vi "Begin.vi"(8 "error in":errorcluster) -> (0 "error out":errorcluster)   [LabVIEW 2018]
doc: "Called before other user functions, this VI is expected to open initial I/O refnums, load in file data, and do all program initialization. Notice that the <B>error out</B> terminal is simply used for data flow. Wiring it to other structures or subVIs ensures that this VI runs first."
uses:
  <vilib>/Rock Robotics/WPI/ThirdParty/Phoenix-LabVIEW/Motor Controller/Controls/CTRE_Phoenix_MotorControl_EnhancedMotorControllerConfigurables.ctl
  <vilib>/Rock Robotics/WPI/ThirdParty/Phoenix-LabVIEW/Motor Controller/Controls/CTRE_Phoenix_MotorControl_BaseConfigurables.ctl
  <vilib>/Rock Robotics/WPI/ThirdParty/Phoenix-LabVIEW/Motor Controller/Controls/CTRE_Phoenix_MotorControl_VelocityMeasurementPeriod.ctl
  <vilib>/Rock Robotics/WPI/ThirdParty/Phoenix-LabVIEW/Motor Controller/Controls/CTRE_Phoenix_MotorControl_SlotStructure.ctl
  <vilib>/Rock Robotics/WPI/ThirdParty/Phoenix-LabVIEW/Motor Controller/Controls/CTRE_Phoenix_MotorControl_FilterStruct.ctl
  <vilib>/Rock Robotics/WPI/ThirdParty/Phoenix-LabVIEW/Motor Controller/Controls/CTRE_Phoenix_MotorControl_RemoteSourceType.ctl
  <vilib>/Rock Robotics/WPI/ThirdParty/Phoenix-LabVIEW/Controls/CTRE_Phoenix_CustomParamConfiguration.ctl
  <vilib>/Rock Robotics/WPI/ThirdParty/Phoenix-LabVIEW/Motor Controller/Controls/CTRE_Phoenix_MotorControl_FeedbackDevice.ctl
  <vilib>/Rock Robotics/WPI/ThirdParty/Phoenix-LabVIEW/Motor Controller/Controls/CTRE_Phoenix_MotorControl_SensorTermFeedbackDevice_Enhanced.ctl
  <vilib>/Rock Robotics/WPI/ThirdParty/Phoenix-LabVIEW/Motor Controller/Controls/CTRE_Phoenix_MotorControl_LimitSwitchNormal.ctl
  <vilib>/Rock Robotics/WPI/ThirdParty/Phoenix-LabVIEW/Motor Controller/Controls/CTRE_Phoenix_MotorControl_LimitSwitchSource_Local.ctl
  <vilib>/Rock Robotics/WPI/ThirdParty/Phoenix-LabVIEW/Motor Controller/Controls/CTRE_Phoenix_MotorControl_MotorControllerConfigurables.ctl
  <vilib>/Rock Robotics/WPI/ThirdParty/Phoenix-LabVIEW/Motor Controller/Controls/CTRE_Phoenix_MotorControl_RemoteFeedbackDevice.ctl
  <vilib>/Rock Robotics/WPI/ThirdParty/Phoenix-LabVIEW/Motor Controller/Controls/CTRE_Phoenix_MotorControl_SensorTermFeedbackDevice.ctl
  <vilib>/Rock Robotics/WPI/ThirdParty/Phoenix-LabVIEW/Motor Controller/Controls/CTRE_Phoenix_MotorControl_LimitSwitchSource.ctl
  <vilib>/Rock Robotics/WPI/DriverStation/WPI_DriverStationRobotMode2.ctl
  <vilib>/Rock Robotics/WPI/Joystick/WPI_JoystickDeviceEnum.ctl
  <vilib>/Rock Robotics/WPI/ThirdParty/REV Robotics/SPARK MAX/Typedef/Spark MAX Idle Mode.ctl
  <vilib>/Rock Robotics/WPI/ThirdParty/Phoenix-LabVIEW/Motor Controller/Controls/CTRE_Phoenix_MotorControl_NeutralMode.ctl
  <vilib>/Rock Robotics/WPI/Solenoid/WPI_SolenoidChannel.ctl
  <vilib>/Rock Robotics/SystemInterfaces/AI/FPGA_AIChannel.ctl
  <vilib>/Rock Robotics/WPI/Accelerometer/WPI_AccelerometerRange.ctl
  Robot Global Data.vi
  <vilib>/Rock Robotics/Network Tables/NT Write String Array.vi
  Joystick RefNum.vi
  RefNums_Actuators.vi
  CurrentMonitoring.vi
  <vilib>/Rock Robotics/WPI/Solenoid/WPI_SolenoidOpenDouble.vi
  <vilib>/Rock Robotics/WPI/Utilities/WPI_GetSetVariantRefNum.vi
  RefNums_Sensors.vi
  <vilib>/Rock Robotics/WPI/Accelerometer/InternalAccelerometer/WPI_AccelerometerInternalOpen.vi
  <vilib>/Rock Robotics/WPI/Solenoid/WPI_SolenoidOpenSingle.vi
  <vilib>/Rock Robotics/SystemInterfaces/DIO/FPGA_DIOPWMChannel.ctl
panel:
  in  "Victor Enhanced Control":T1={"Base Configurables"={"openLoopRamp"=0.0, "closedLoopRamp"=0.0, "peakOutputForward"=1.0, "peakOutputReverse"=-1.0, "nominalOutputForward"=0.0, "nominalOutputReverse"=0.0, "neutralDeadband"=0.04, "voltageCompSaturation"=0.0, "voltageMeasurementFilter"=32, "velocityMeasurementPeriod"=100, "velocityMeasurementWindow"=64, "forwardSoftLimitThreshold"=0, "reverseSoftLimitThreshold"=0, "forwardSoftLimitEnable"=FALSE, "reverseSoftLimitEnable"=FALSE, "slot0"={"P"=0.0, "I"=0.0, "D"=0.0, "F"=0.0, "integralZone"=0.0, "allowableClosedLoopError"=0, "maxIntegralAccumulator"=0.0, "closedLoopPeakOutput"=1.0, "closedLoopPeriod"=1}, "slot1"={"P"=0.0, "I"=0.0, "D"=0.0, "F"=0.0, "integralZone"=0.0, "allowableClosedLoopError"=0, "maxIntegralAccumulator"=0.0, "closedLoopPeakOutput"=1.0, "closedLoopPeriod"=1}, "slot2"={"P"=0.0, "I"=0.0, "D"=0.0, "F"=0.0, "integralZone"=0.0, "allowableClosedLoopError"=0, "maxIntegralAccumulator"=0.0, "closedLoopPeakOutput"=1.0, "closedLoopPeriod"=1}, "slot3"={"P"=0.0, "I"=0.0, "D"=0.0, "F"=0.0, "integralZone"=0.0, "allowableClosedLoopError"=0, "maxIntegralAccumulator"=0.0, "closedLoopPeakOutput"=1.0, "closedLoopPeriod"=1}, "auxPIDPolarity"=FALSE, "remoteFilter0"={"remoteSensorDeviceID"=0, "remoteSensorSource"=enum."Off"}, "remoteFilter1"={"remoteSensorDeviceID"=0, "remoteSensorSource"=enum."Off"}, "motionCruiseVelocity"=0, "motionAcceleration"=0, "motionProfileTrajectoryPeriod"=0, "feedbackNotContinuous"=FALSE, "remoteSensorClosedLoopDisableNeutralOnLOS"=FALSE, "clearPositionOnLimitF"=FALSE, "clearPositionOnLimitR"=FALSE, "clearPositionOnQuadIdx"=FALSE, "limitSwitchDisableNeutralOnLOS"=FALSE, "softLimitDisableNeutralOnLOS"=FALSE, "pulseWidthPeriod_EdgesPerRot"=1, "pulseWidthPeriod_FilterWindowSz"=1, "customParam"={"customParam0"=0, "customParam1"=0}, "trajectoryInterpolationEnable"=TRUE}, "primaryPID"={"selectedFeedbackCoefficient"=1.0, "selectedFeedbackSensor"=11}, "auxiliaryPID"={"selectedFeedbackCoefficient"=1.0, "selectedFeedbackSensor"=11}, "sum 0 term"=11, "sum 1 term"=11, "diff 0 term "=11, "diff 1 term"=11, "forwardLimitSwitchDeviceID"=0, "reverseLimitSwitchDeviceID"=0, "forwardLimitSwitchNormal"=enum."Normally Open", "reverseLimitSwitchNormal"=enum."Normally Open", "forwardLimitSwitchSource"=3, "reverseLimitSwitchSource"=3} {"diff 1 term" items=["Remote Source 0"=11, "Remote Source 1"=12, "Software Emulated"=15]; "diff 0 term" items=["Remote Source 0"=11, "Remote Source 1"=12, "Software Emulated"=15]; "sum 1 term" items=["Remote Source 0"=11, "Remote Source 1"=12, "Software Emulated"=15]; "sum 0 term" items=["Remote Source 0"=11, "Remote Source 1"=12, "Software Emulated"=15]; "reverseLimitSwitchSource" items=["Remote Talon SRX"=1, "Remote CANifier"=2, "Deactivated"=3]; "forwardLimitSwitchSource" items=["Remote Talon SRX"=1, "Remote CANifier"=2, "Deactivated"=3]; "auxiliaryPID"."selectedFeedbackSensor" items=["Sensor Sum (S0 + S1)"=9, "Sensor Difference (D0 - D1)"=10, "Remote Source 0"=11, "Remote Source 1"=12, "Software Emulated"=15]; "primaryPID"."selectedFeedbackSensor" items=["Sensor Sum (S0 + S1)"=9, "Sensor Difference (D0 - D1)"=10, "Remote Source 0"=11, "Remote Source 1"=12, "Software Emulated"=15]; "Base Configurables"."velocityMeasurementPeriod" items=["Period_1ms"=1, "Period_2ms"=2, "Period_5ms"=5, "Period_10ms"=10, "Period_20ms"=20, "Period_25ms"=25, "Period_50ms"=50, "Period_100ms"=100]}
  in  "Talon Enhanced Config":T12={"Base Configurables"={"openLoopRamp"=0.0, "closedLoopRamp"=0.0, "peakOutputForward"=1.0, "peakOutputReverse"=-1.0, "nominalOutputForward"=0.0, "nominalOutputReverse"=0.0, "neutralDeadband"=0.04, "voltageCompSaturation"=0.0, "voltageMeasurementFilter"=32, "velocityMeasurementPeriod"=100, "velocityMeasurementWindow"=64, "forwardSoftLimitThreshold"=0, "reverseSoftLimitThreshold"=0, "forwardSoftLimitEnable"=FALSE, "reverseSoftLimitEnable"=FALSE, "slot0"={"P"=0.0, "I"=0.0, "D"=0.0, "F"=0.0, "integralZone"=0.0, "allowableClosedLoopError"=0, "maxIntegralAccumulator"=0.0, "closedLoopPeakOutput"=1.0, "closedLoopPeriod"=1}, "slot1"={"P"=0.0, "I"=0.0, "D"=0.0, "F"=0.0, "integralZone"=0.0, "allowableClosedLoopError"=0, "maxIntegralAccumulator"=0.0, "closedLoopPeakOutput"=1.0, "closedLoopPeriod"=1}, "slot2"={"P"=0.0, "I"=0.0, "D"=0.0, "F"=0.0, "integralZone"=0.0, "allowableClosedLoopError"=0, "maxIntegralAccumulator"=0.0, "closedLoopPeakOutput"=1.0, "closedLoopPeriod"=1}, "slot3"={"P"=0.0, "I"=0.0, "D"=0.0, "F"=0.0, "integralZone"=0.0, "allowableClosedLoopError"=0, "maxIntegralAccumulator"=0.0, "closedLoopPeakOutput"=1.0, "closedLoopPeriod"=1}, "auxPIDPolarity"=FALSE, "remoteFilter0"={"remoteSensorDeviceID"=0, "remoteSensorSource"=enum."Off"}, "remoteFilter1"={"remoteSensorDeviceID"=0, "remoteSensorSource"=enum."Off"}, "motionCruiseVelocity"=0, "motionAcceleration"=0, "motionProfileTrajectoryPeriod"=0, "feedbackNotContinuous"=FALSE, "remoteSensorClosedLoopDisableNeutralOnLOS"=FALSE, "clearPositionOnLimitF"=FALSE, "clearPositionOnLimitR"=FALSE, "clearPositionOnQuadIdx"=FALSE, "limitSwitchDisableNeutralOnLOS"=FALSE, "softLimitDisableNeutralOnLOS"=FALSE, "pulseWidthPeriod_EdgesPerRot"=1, "pulseWidthPeriod_FilterWindowSz"=1, "customParam"={"customParam0"=0, "customParam1"=0}, "trajectoryInterpolationEnable"=TRUE}, "primaryPID"={"selectedFeedbackCoefficient"=1.0, "selectedFeedbackSensor"=0}, "auxiliaryPID"={"selectedFeedbackCoefficient"=1.0, "selectedFeedbackSensor"=0}, "sum0Term"=0, "sum1Term"=0, "diff0Term"=0, "diff1Term"=0, "forwardLimitSwitchNormal"=enum."Normally Open", "reverseLimitSwitchNormal"=enum."Normally Open", "forwardLimitSwitchDeviceID"=0, "reverseLimitSwitchDeviceID"=0, "forwardLimitSwitchSource"=enum."Feedback Connector", "reverseLimitSwitchSource"=enum."Feedback Connector", "peakCurrentLimit"=1, "peakCurrentDuration"=1, "continuousCurrentLimit"=1} {"diff1Term" items=["QuadEncoder"=0, "Analog"=2, "Tachometer"=4, "Pulse Width Encoded Position"=8, "Remote Source 0"=11, "Remote Source 1"=12, "Software Emulated"=15]; "diff0Term" items=["QuadEncoder"=0, "Analog"=2, "Tachometer"=4, "Pulse Width Encoded Position"=8, "Remote Source 0"=11, "Remote Source 1"=12, "Software Emulated"=15]; "sum1Term" items=["QuadEncoder"=0, "Analog"=2, "Tachometer"=4, "Pulse Width Encoded Position"=8, "Remote Source 0"=11, "Remote Source 1"=12, "Software Emulated"=15]; "sum0Term" items=["QuadEncoder"=0, "Analog"=2, "Tachometer"=4, "Pulse Width Encoded Position"=8, "Remote Source 0"=11, "Remote Source 1"=12, "Software Emulated"=15]; "auxiliaryPID"."selectedFeedbackSensor" items=["QuadEncoder"=0, "Analog"=2, "Tachometer"=4, "Pulse Width Encoded Position"=8, "Sensor Sum (S0 + S1)"=9, "Sensor Difference (D0 - D1)"=10, "Remote Source 0"=11, "Remote Source 1"=12, "Software Emulated"=15]; "primaryPID"."selectedFeedbackSensor" items=["QuadEncoder"=0, "Analog"=2, "Tachometer"=4, "Pulse Width Encoded Position"=8, "Sensor Sum (S0 + S1)"=9, "Sensor Difference (D0 - D1)"=10, "Remote Source 0"=11, "Remote Source 1"=12, "Software Emulated"=15]; "Base Configurables"."velocityMeasurementPeriod" items=["Period_1ms"=1, "Period_2ms"=2, "Period_5ms"=5, "Period_10ms"=10, "Period_20ms"=20, "Period_25ms"=25, "Period_50ms"=50, "Period_100ms"=100]}
  # "Sum and Diff terms are ways to select more than one sensor as a feedback device. \n Sum 0 is the first feedback device to be used for the Sum term, \n Sum 1 is the feedback device to be added to Sum 0 for the Sum term\n Diff 0 and Diff 1 work in a similar manner"
  # "These are only applicable\nif using a remote limit switch.\n\nLocal limit switches/no limit\nswitches do not use this"
  # "False: Primary Output = PID[0] + PID[1]  ---  Auxiliary Output = PID[0] - PID[1]\nTrue:  Primary Output = PID[0] - PID[1] --- Auxiliary Output = PID[0] + PID[1]"
  # "Enable the motion profile executor to perform linear interpolation between profile points.  Defaults to True."
  # "Sum and Diff terms are ways to select more than one sensor as a feedback device. \n Sum 0 is the first feedback device to be used for the Sum term.\n Sum 1 is the feedback device to be added to Sum 0 for the Sum term.\n Diff 0 and Diff 1 work in a similar manner."
  # "These are only applicable\nif using a remote limit switch.\n\nLocal limit switches/no limit\nswitches do not use this."
  # "Current is below Continuous threshold AND\n\n(Requested output is weaker** than applied motor\noutput OR is in the opposite direction).\n/\nMotor output is set to requested output."
  # "Current is above Peak* Threshold for Peak Duration.\n/\nReduce motor output (towards neutral)."
  # "Current is below Continuous threshold.\n/\nRamp motor output towards requested output."
  # "Current is above Continuous threshold.\n/\nReduce motor output (towards neutral)."
  # "Current Limiting is NOT enabled\nby default.\nCall this VI to enable."
  # "*If the configured Peak Threshold is less than the Continuous Threshold, the applied Peak Threshold is set equal to the Configured Continuous Threshold in firmware.\n** Both requested output and applied motor output are in the same direction, and requested output is closer to neutral."
  # "False: Primary Output = PID[0] + PID[1]  ---  Auxiliary Output = PID[0] - PID[1]\nTrue:  Primary Output = PID[0] - PID[1] --- Auxiliary Output = PID[0] + PID[1]"
  # "Enable the motion profile executor to perform linear interpolation between profile points.  Defaults to True."
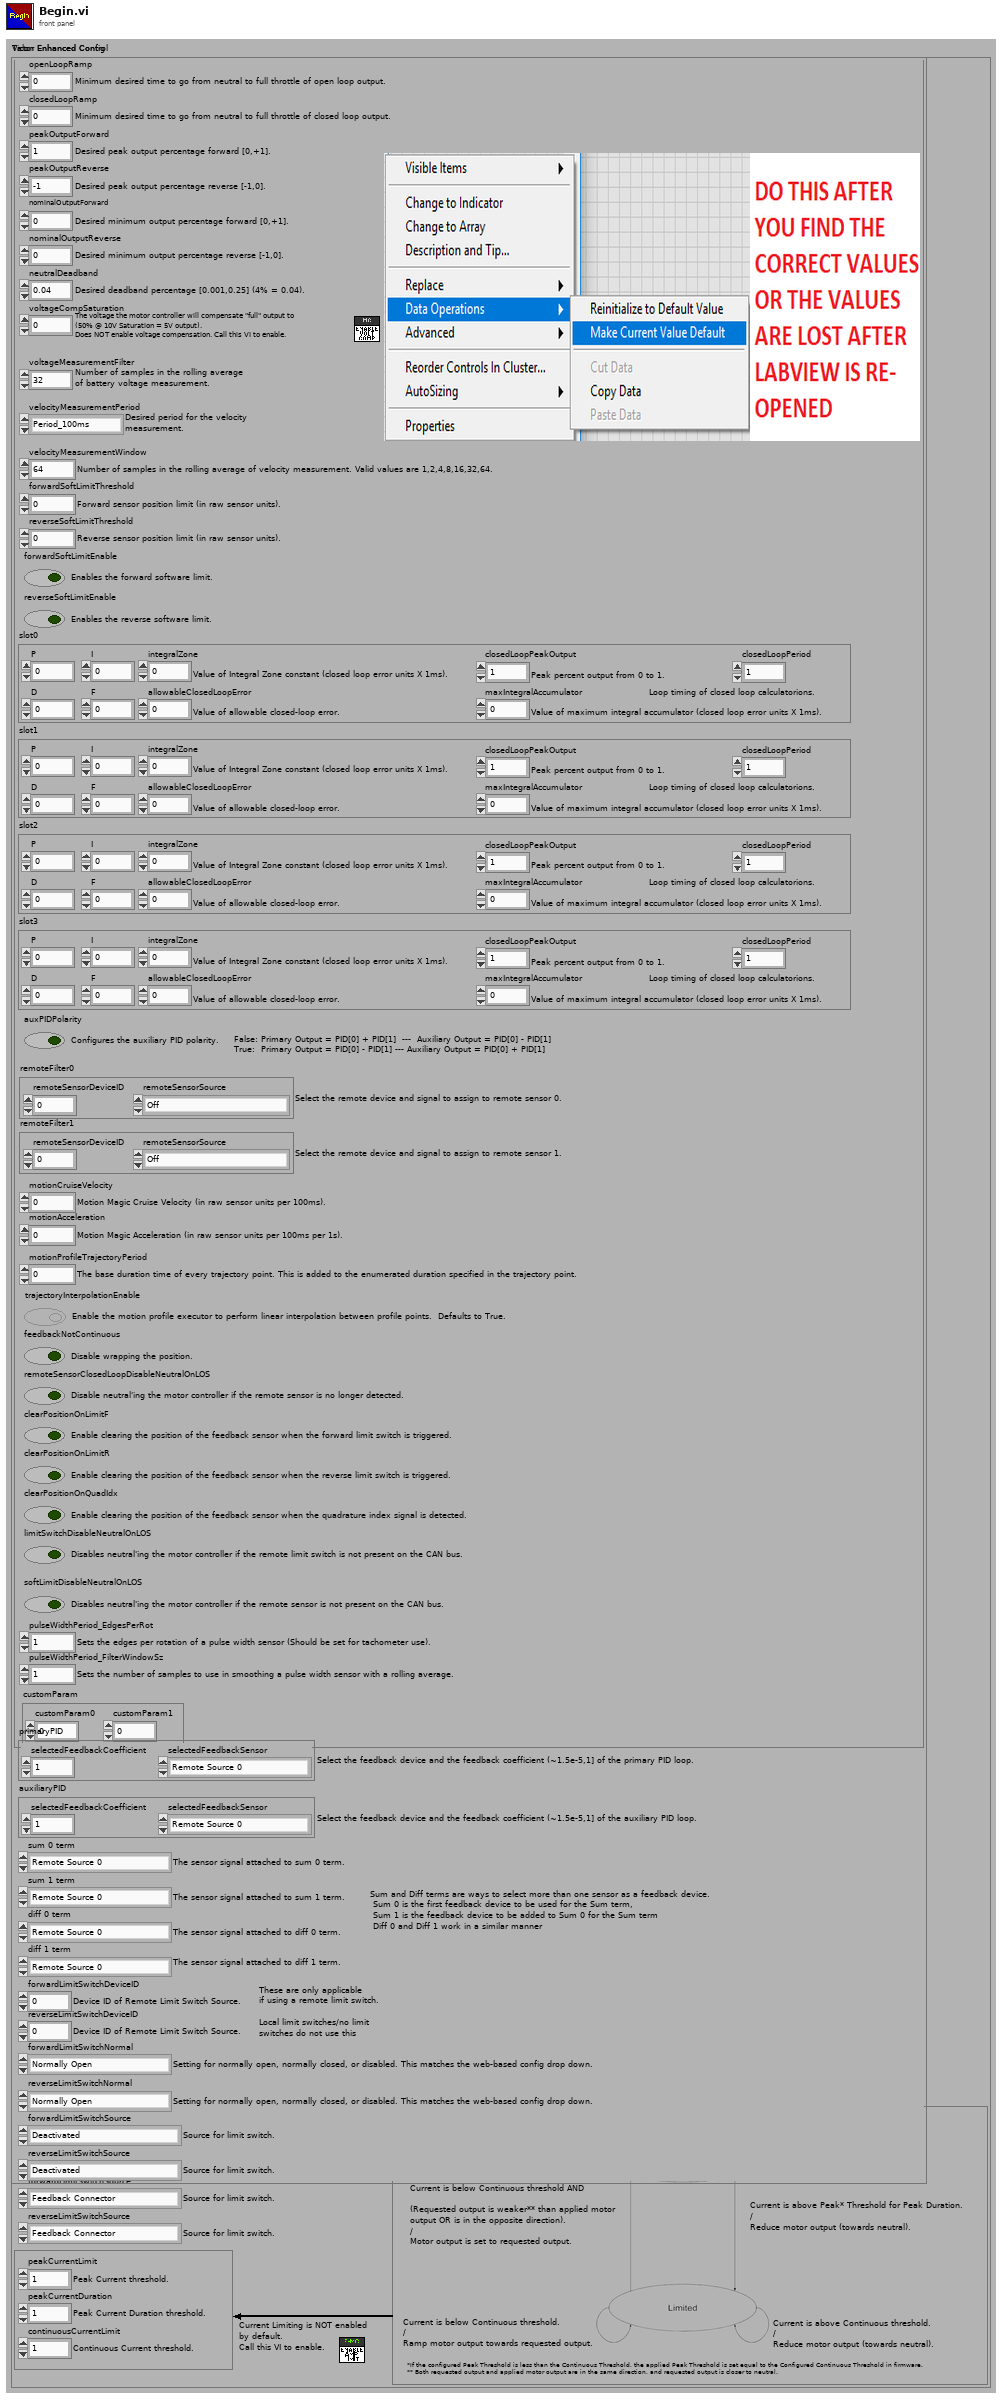
[diagram p1: front panel]
types:
  T1 = typedef "CTRE_Phoenix_MotorControl_MotorControllerConfigurables.ctl" = cluster{"Base Configurables":T2, "primaryPID":cluster{"selectedFeedbackCoefficient":dbl, "selectedFeedbackSensor":T8}, "auxiliaryPID":cluster{"selectedFeedbackCoefficient":dbl, "selectedFeedbackSensor":T8}, "sum 0 term":T9, "sum 1 term":T9, "diff 0 term ":T9, "diff 1 term":T9, "forwardLimitSwitchDeviceID":i32, "reverseLimitSwitchDeviceID":i32, "forwardLimitSwitchNormal":T10, "reverseLimitSwitchNormal":T10, "forwardLimitSwitchSource":T11, "reverseLimitSwitchSource":T11}
  T2 = typedef "CTRE_Phoenix_MotorControl_BaseConfigurables.ctl" = cluster{"openLoopRamp":dbl, "closedLoopRamp":dbl, "peakOutputForward":dbl, "peakOutputReverse":dbl, "nominalOutputForward":dbl, "nominalOutputReverse":dbl, "neutralDeadband":dbl, "voltageCompSaturation":dbl, "voltageMeasurementFilter":i32, "velocityMeasurementPeriod":T3, "velocityMeasurementWindow":i32, "forwardSoftLimitThreshold":i32, "reverseSoftLimitThreshold":i32, "forwardSoftLimitEnable":bool, "reverseSoftLimitEnable":bool, "slot0":T4, "slot1":T4, "slot2":T4, "slot3":T4, "auxPIDPolarity":bool, "remoteFilter0":T5, "remoteFilter1":T5, "motionCruiseVelocity":i32, "motionAcceleration":i32, "motionProfileTrajectoryPeriod":i32, "feedbackNotContinuous":bool, "remoteSensorClosedLoopDisableNeutralOnLOS":bool, "clearPositionOnLimitF":bool, "clearPositionOnLimitR":bool, "clearPositionOnQuadIdx":bool, "limitSwitchDisableNeutralOnLOS":bool, "softLimitDisableNeutralOnLOS":bool, "pulseWidthPeriod_EdgesPerRot":i32, "pulseWidthPeriod_FilterWindowSz":i32, "customParam":T7, "trajectoryInterpolationEnable":bool}
  T3 = typedef "CTRE_Phoenix_MotorControl_VelocityMeasurementPeriod.ctl" = u16
  T4 = typedef "CTRE_Phoenix_MotorControl_SlotStructure.ctl" = cluster{"P":dbl, "I":dbl, "D":dbl, "F":dbl, "integralZone":dbl, "allowableClosedLoopError":i32, "maxIntegralAccumulator":dbl, "closedLoopPeakOutput":dbl, "closedLoopPeriod":i32}
  T5 = typedef "CTRE_Phoenix_MotorControl_FilterStruct.ctl" = cluster{"remoteSensorDeviceID":u8, "remoteSensorSource":T6}
  T6 = typedef "CTRE_Phoenix_MotorControl_RemoteSourceType.ctl" = enum16{"Off", "Talon SRX Selected Sensor", "Pigeon IMU Yaw", "Pigeon IMU Pitch", "Pigeon IMU Roll", "CANifier Quadrature", "CANifier PWM Input 0", "CANifier PWM Input 1", "CANifier PWM Input 2", "CANifier PWM Input 3", "Gadgeteer Pigeon Yaw", "Gadgeteer Pigeon Pitch", "Gadgeteer Pigeon Roll"}
  T7 = typedef "CTRE_Phoenix_CustomParamConfiguration.ctl" = cluster{"customParam0":i32, "customParam1":i32}
  T8 = typedef "CTRE_Phoenix_MotorControl_RemoteFeedbackDevice.ctl" = i8
  T9 = typedef "CTRE_Phoenix_MotorControl_SensorTermFeedbackDevice.ctl" = i8
  T10 = typedef "CTRE_Phoenix_MotorControl_LimitSwitchNormal.ctl" = enum16{"Normally Open", "Normally Closed", "Disabled"}
  T11 = typedef "CTRE_Phoenix_MotorControl_LimitSwitchSource.ctl" = u16
  T12 = typedef "CTRE_Phoenix_MotorControl_EnhancedMotorControllerConfigurables.ctl" = cluster{"Base Configurables":T2, "primaryPID":cluster{"selectedFeedbackCoefficient":dbl, "selectedFeedbackSensor":T13}, "auxiliaryPID":cluster{"selectedFeedbackCoefficient":dbl, "selectedFeedbackSensor":T13}, "sum0Term":T14, "sum1Term":T14, "diff0Term":T14, "diff1Term":T14, "forwardLimitSwitchNormal":T10, "reverseLimitSwitchNormal":T10, "forwardLimitSwitchDeviceID":i32, "reverseLimitSwitchDeviceID":i32, "forwardLimitSwitchSource":T15, "reverseLimitSwitchSource":T15, "peakCurrentLimit":i32, "peakCurrentDuration":i32, "continuousCurrentLimit":i32}
  T13 = typedef "CTRE_Phoenix_MotorControl_FeedbackDevice.ctl" = i8
  T14 = typedef "CTRE_Phoenix_MotorControl_SensorTermFeedbackDevice_Enhanced.ctl" = i8
  T15 = typedef "CTRE_Phoenix_MotorControl_LimitSwitchSource_Local.ctl" = enum16{"Feedback Connector", "Remote Talon SRX", "Remote CANifier", "Deactivated"}
  T16 = typedef "WPI_AccelerometerRange.ctl" = enum16{"+/- 2 g", "+/- 4 g", "+/- 8 g"}
  T17 = typedef "FPGA_AIChannel.ctl" = enum8{"AI 0", "AI 1", "AI 2", "AI 3", "AI MXP 0", "AI MXP 1", "AI MXP 2", "AI MXP 3", "Invalid"}
  T18 = typedef "WPI_SolenoidChannel.ctl" = enum8{"Solenoid 0", "Solenoid 1", "Solenoid 2", "Solenoid 3", "Solenoid 4", "Solenoid 5", "Solenoid 6", "Solenoid 7", "Invalid"}
  T19 = typedef "CTRE_Phoenix_MotorControl_NeutralMode.ctl" = enum8{"EEPROMSetting", "Override to Coast", "Override to Brake"}
  T20 = typedef "Spark MAX Idle Mode.ctl" = enum16{"Coast", "Brake"}
  T21 = typedef "WPI_JoystickDeviceEnum.ctl" = enum16{"USB 0", "USB 1", "USB 2", "USB 3", "USB 4", "USB 5"}
  T22 = typedef "WPI_DriverStationRobotMode2.ctl" = enum16{"Autonomous Disabled", "Autonomous Enabled", "Teleop Disabled", "Teleop Enabled", "Disconnected", "Finish", "Test Disabled", "Test Enabled", "Emergency Stopped"}
  T23 = typedef "WPI_MotorControlDeviceRef.ctl" = cluster{"DeviceStatus":errorcluster, "Type":T24, "PWM":cluster{"PWM Channel":T25, "DeadBand":T26}, "CAN":cluster{"Device Number":u8, "SetOutput VI Ref":variant, "GetOutput VI Ref":variant, "Enable VI Ref":variant, "Disable VI Ref":variant, "Data":variant}, "Invert":bool, "DIO PWM":cluster{"PWM \"Enable\" Channel":T25, "DIOChannel":T27, "PWM Rate":dbl}}
  T24 = typedef "WPI_MotorControlType.ctl" = enum16{"PWM", "CAN", "DIO PWM"}
  T25 = typedef "FPGA_DIOPWMChannel.ctl" = enum8{"PWM 0", "PWM 1", "PWM 2", "PWM 3", "PWM 4", "PWM 5", "PWM 6", "PWM 7", "PWM 8", "PWM 9", "PWM MXP 0", "PWM MXP 1", "PWM MXP 2", "PWM MXP 3", "PWM MXP 4", "PWM MXP 5", "PWM MXP 6", "PWM MXP 7", "PWM MXP 8", "PWM MXP 9", "Invalid"}
  T26 = typedef "WPI_PWMDeadband.ctl" = cluster{"Name":string, "maxPositivePwm":i32, "minPositivePwm":i32, "centerPwm":i32, "maxNegativePwm":i32, "minNegativePwm":i32, "angularRange":u16}
  T27 = typedef "FPGA_DIOChannel.ctl" = enum8{"DIO 0", "DIO 1", "DIO 2", "DIO 3", "DIO 4", "DIO 5", "DIO 6", "DIO 7", "DIO 8", "DIO 9", "DIO MXP 0", "DIO MXP 1", "DIO MXP 2", "DIO MXP 3", "DIO MXP 4", "DIO MXP 5", "DIO MXP 6", "DIO MXP 7", "DIO MXP 8", "DIO MXP 9", "DIO MXP 10", "DIO MXP 11", "DIO MXP 12", "DIO MXP 13", "DIO MXP 14", "DIO MXP 15", "SPI Port CS1", "SPI Port CS2", "SPI Port CS3", "SPI Port MISO", "SPI Port MOSI", "Invalid"}
  T28 = typedef "WPI_ServoDeviceRef.ctl" = cluster{"DeviceStatus":errorcluster, "PWM Channel":T25, "DeadBand":T26}
  T29 = typedef "WPI_JoystickDevRef.ctl" = cluster{"Device":T21}
  T30 = typedef "WPI_SolenoidDevRef.ctl" = cluster{"DevStatus":errorcluster, "Pneumatics Control Module":u8, "Forward Solenoid Channel":T18, "Reverse Solenoid Channel":T18}
  T31 = typedef "WPI_CompressorDevRef.ctl" = cluster{"DevStatus":errorcluster, "Pneumatics Control Module":u8}
  T32 = typedef "WPI_AnalogChannelDevRef.ctl" = cluster{"DevStatus":errorcluster, "Analog Channel":T17}
  T33 = typedef "WPI_AccelerometerDevRef.ctl" = cluster{"DevStatus":errorcluster, "Scaling":T34, "Analog Channels":T35, "I2C Bus":T36, "SPI Bus":T37, "Accel Range":T38, "ADXL Axes":T39, "Handle":i32, "Device Address":u8, "Accel Type":enum16{"Analog", "ADXL345 I2C", "ADXL345 SPI", "Internal", "ADXL362 SPI"}}
  T34 = typedef "WPI_AccelerometerScaling.ctl" = cluster{"Gain (VoltsPerG)":dbl, "Center Voltage":dbl}
  T35 = typedef "WPI_AccelerometerAnalogChannels.ctl" = cluster{"X-Axis":T17, "Y-Axis":T17, "Z-Axis":T17}
  T36 = typedef "i2c_bus.ctl" = enum16{"I2C On-Board", "I2C MXP", "Invalid"}
  T37 = typedef "spi_bus.ctl" = enum16{"SPI On-Board, CS0", "SPI On-Board, CS1", "SPI On-Board, CS2", "SPI On-Board, CS3", "SPI MXP", "Invalid"}
  T38 = typedef "ADXL345 Range.ctl" = u8
  T39 = typedef "WPI_AccelerometerADXL345 Axes.ctl" = cluster{"X-Axis":bool, "Y-Axis":bool, "Z-Axis":bool}
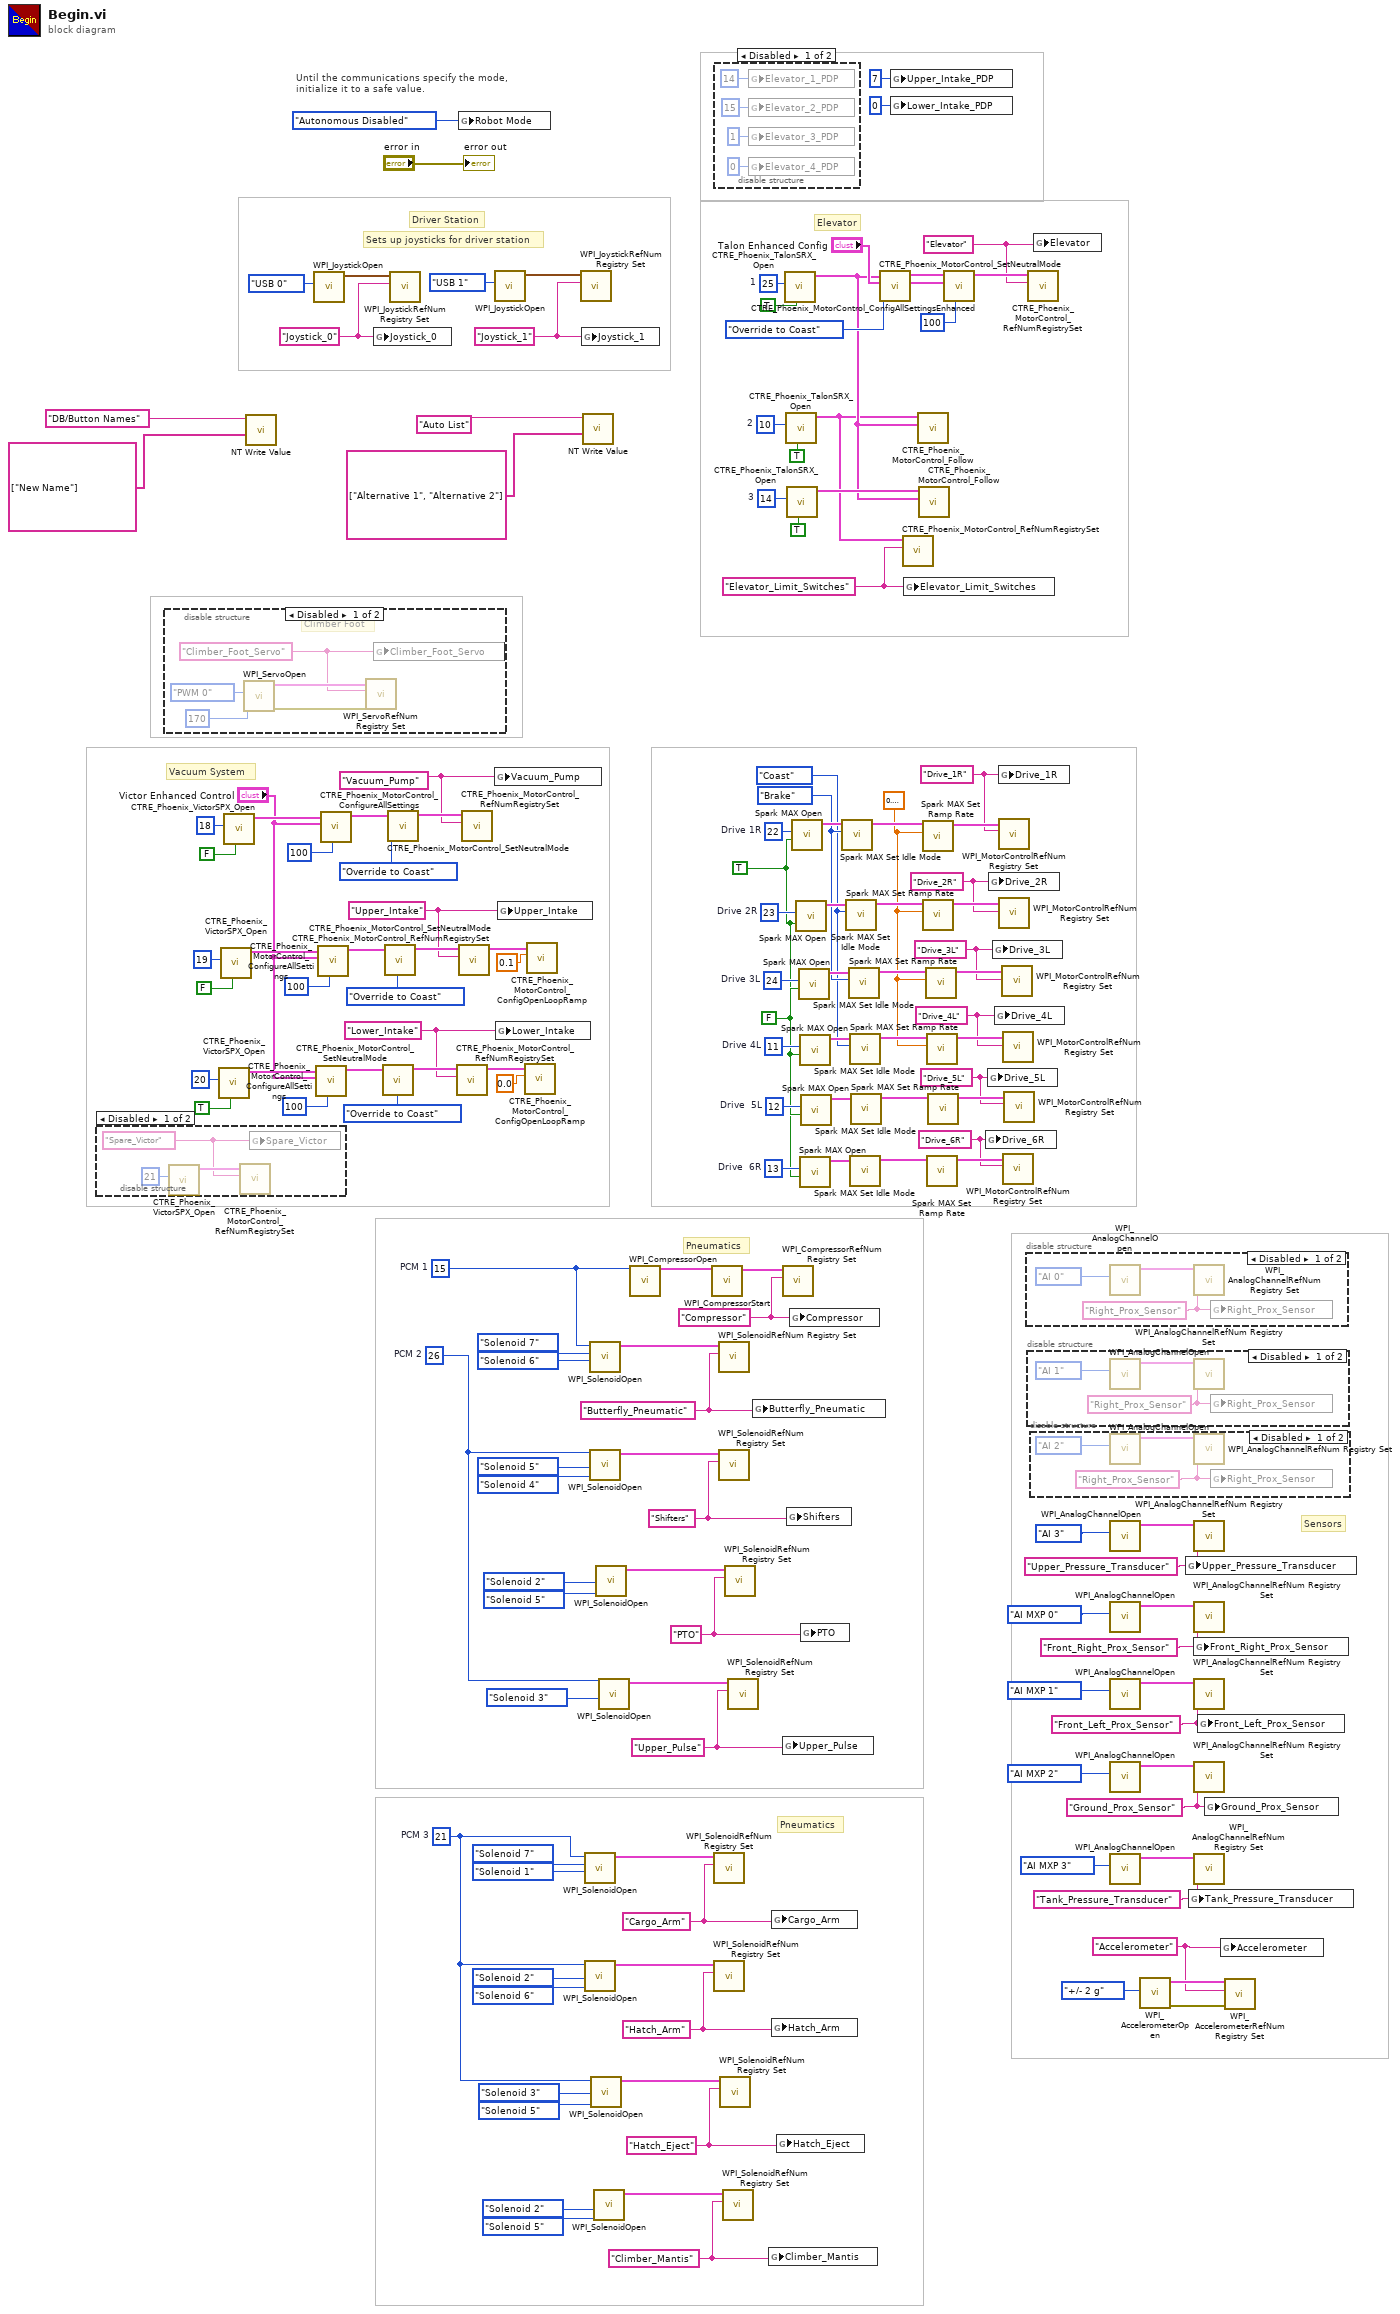
[diagram p0: block diagram]
diagram:
  w2 = u8 26  # PCM 2
  w3 = "Accelerometer" ("refnum name")
  w7 = "Tank_Pressure_Transducer" ("refnum name")
  w10 = "Ground_Prox_Sensor" ("refnum name")
  w13 = "Front_Left_Prox_Sensor" ("refnum name")
  w16 = "Front_Right_Prox_Sensor" ("refnum name")
  w19 = "Upper_Pressure_Transducer" ("refnum name")
  w22 = u8 21  # PCM 3
  w26 = "Climber_Mantis" ("refnum name")
  w29 = "Hatch_Eject" ("refnum name")
  w33 = "Hatch_Arm" ("refnum name")
  w35 = "Cargo_Arm" ("refnum name")
  w41 = "Upper_Pulse" ("refnum name")
  w44 = "PTO" ("refnum name")
  w48 = "Shifters" ("refnum name")
  w50 = "Compressor" ("refnum name")
  w51 = "Butterfly_Pneumatic" ("refnum name")
  w1 = u8 15  # PCM 1
  w59 = "Lower_Intake" ("refnum name")
  w64 = "Upper_Intake" ("refnum name")
  w78 = "Vacuum_Pump" ("refnum name")
  w86 = "Elevator_Limit_Switches" ("refnum name")
  w91 = u8 14  # 3
  w93 = u8 10  # 2
  w99 = "Elevator" ("refnum name")
  w103 = u8 25  # 1
  w105 = "Drive_6R" ("refnum name")
  w108 = u8 13  # Drive  6R
  w104 = "Drive_5L" ("refnum name")
  w113 = u8 12  # Drive  5L
  w118 = "Drive_4L" ("refnum name")
  w120 = u8 11  # Drive 4L
  w111 = FALSE ("Invert")
  w123 = "Drive_3L" ("refnum name")
  w126 = u8 24  # Drive 3L
  w129 = "Drive_2R" ("refnum name")
  w116 = Spark_MAX_Idle_Mode."Coast" ("Idle Mode")
  w131 = u8 23  # Drive 2R
  w134 = "Drive_1R" ("refnum name")
  w117 = sgl 0.1 ("Seconds from neutral to full (0)")
  w124 = Spark_MAX_Idle_Mode."Brake" ("Idle Mode")
  w106 = TRUE ("Invert")
  w135 = u8 22  # Drive 1R
  w141 = "Joystick_1" ("Joystick_1")
  w142 = "Joystick_0" ("Joystick_0")
  # "Sensors"
  # "Pneumatics"
  # "Pneumatics"
  # "Vacuum System"
  # "Elevator"
  # "Sets up joysticks for driver station"
  # "Driver Station"
  # "Until the communications specify the mode,\ninitialize it to a safe value."
  n1 = disable-structure shown="Disabled" {
    frame Disabled {
      w151 = "Spare_Victor" ("refnum name")
      n2 = call <vilib>:"CTRE_Phoenix_VictorSPX_Open.vi"("Device Number"=u8 21) -> ("CAN Talon SRX Ref"=w152:T23)  [unwired: 9 in, 1 out]
      n3 = call <vilib>:"CTRE_Phoenix_MotorControl_RefNumRegistrySet.vi"("refnum name"=w151, "PhoenixMotorControlDevRef"=w152) -> ()  [unwired: 8 in, 2 out]
      n4 = global write "RefNums_Actuators.vi" "Spare_Victor"(w151) -> ()
    }
    frame Enabled {
    }
  }
  n5 = disable-structure shown="Disabled" {
    frame Disabled {
      w154 = "Climber_Foot_Servo" ("refnum name")
      # "Climber Foot"
      n6 = call <vilib>:"WPI_ServoOpen.vi"("Angular Range"=u16 170, "PWM Channel"=FPGA_DIOPWMChannel."PWM 0") -> ("error out"=w155:errorcluster, "ServoDeviceRef"=w158:T28)  [unwired: 8 in]
      n7 = call <vilib>:"WPI_ServoRefNum Registry Set.vi"("error in (no error)"=w155, "refnum name"=w154, "ServoDeviceRef"=w158) -> ()  [unwired: 7 in, 2 out]
      n8 = global write "RefNums_Actuators.vi" "Climber_Foot_Servo"(w154) -> ()
    }
    frame Enabled {
    }
  }
  n9 = call <vilib>:"CTRE_Phoenix_VictorSPX_Open.vi"("Invert"=TRUE, "Device Number"=u8 20) -> ("CAN Talon SRX Ref"=w69:T23)  [unwired: 8 in, 1 out]
  n10 = call <vilib>:"CTRE_Phoenix_VictorSPX_Open.vi"("Invert"=FALSE, "Device Number"=u8 19) -> ("CAN Talon SRX Ref"=w75:T23)  [unwired: 8 in, 1 out]
  n11 = call <vilib>:"CTRE_Phoenix_VictorSPX_Open.vi"("Invert"=FALSE, "Device Number"=u8 18) -> ("CAN Talon SRX Ref"=w83:T23)  [unwired: 8 in, 1 out]
  n12 = call-poly <vilib>:"NT Write Value.vi"("String Array"=string[] ["New Name"], "Name"="DB/Button Names") -> ()  [unwired: 9 in, 1 out]
  n13 = call <vilib>:"WPI_JoystickOpen.vi"("JoystickDevice"=WPI_JoystickDeviceEnum."USB 0") -> ("JoystickDevRef"=w143:T29)  [unwired: 10 in]
  n14 = call <vilib>:"CTRE_Phoenix_MotorControl_ConfigureAllSettings.vi"("timeoutMs"=100, "Motor Controller Configurables"="Victor Enhanced Control", "PhoenixMotorControlDevRef"=w69) -> ("PhoenixMotorControlDevRef"=w67:T23)  [unwired: 7 in, 1 out]
  n15 = call <vilib>:"CTRE_Phoenix_MotorControl_ConfigureAllSettings.vi"("timeoutMs"=100, "Motor Controller Configurables"="Victor Enhanced Control", "PhoenixMotorControlDevRef"=w75) -> ("PhoenixMotorControlDevRef"=w73:T23)  [unwired: 7 in, 1 out]
  n16 = call <vilib>:"CTRE_Phoenix_MotorControl_ConfigureAllSettings.vi"("timeoutMs"=100, "Motor Controller Configurables"="Victor Enhanced Control", "PhoenixMotorControlDevRef"=w83) -> ("PhoenixMotorControlDevRef"=w81:T23)  [unwired: 7 in, 1 out]
  n17 = global write "Joystick RefNum.vi" "Joystick_0"(w142) -> ()
  n18 = call <vilib>:"CTRE_Phoenix_MotorControl_SetNeutralMode.vi"("Motor Control Neutral Mode"=CTRE_Phoenix_MotorControl_NeutralMode."Override to Coast", "PhoenixMotorControlDevRef"=w67) -> ("PhoenixMotorControlDevRef"=w66:T23)  [unwired: 8 in, 1 out]
  n19 = call <vilib>:"CTRE_Phoenix_MotorControl_SetNeutralMode.vi"("Motor Control Neutral Mode"=CTRE_Phoenix_MotorControl_NeutralMode."Override to Coast", "PhoenixMotorControlDevRef"=w73) -> ("PhoenixMotorControlDevRef"=w72:T23)  [unwired: 8 in, 1 out]
  n20 = call <vilib>:"CTRE_Phoenix_MotorControl_SetNeutralMode.vi"("Motor Control Neutral Mode"=CTRE_Phoenix_MotorControl_NeutralMode."Override to Coast", "PhoenixMotorControlDevRef"=w81) -> ("PhoenixMotorControlDevRef"=w80:T23)  [unwired: 8 in, 1 out]
  n21 = call <vilib>:"WPI_JoystickRefNum Registry Set.vi"("refnum name"=w142, "JoystickDevRef"=w143) -> ()  [unwired: 8 in, 2 out]
  n22 = call <vilib>:"CTRE_Phoenix_MotorControl_RefNumRegistrySet.vi"("refnum name"=w59, "PhoenixMotorControlDevRef"=w66) -> ("PhoenixMotorControlDevRef"=w62:T23)  [unwired: 8 in, 1 out]
  n23 = global write "Robot Global Data.vi" "Robot Mode"(WPI_DriverStationRobotMode2."Autonomous Disabled" ("Robot Mode")) -> ()
  n24 = call <vilib>:"CTRE_Phoenix_MotorControl_RefNumRegistrySet.vi"("refnum name"=w64, "PhoenixMotorControlDevRef"=w72) -> ("PhoenixMotorControlDevRef"=w63:T23)  [unwired: 8 in, 1 out]
  n25 = call <vilib>:"CTRE_Phoenix_MotorControl_RefNumRegistrySet.vi"("refnum name"=w78, "PhoenixMotorControlDevRef"=w80) -> ()  [unwired: 8 in, 2 out]
  n26 = call <vilib>:"WPI_JoystickOpen.vi"("JoystickDevice"=WPI_JoystickDeviceEnum."USB 1") -> ("JoystickDevRef"=w140:T29)  [unwired: 10 in]
  n27 = global write "RefNums_Actuators.vi" "Vacuum_Pump"(w78) -> ()
  n28 = global write "RefNums_Actuators.vi" "Lower_Intake"(w59) -> ()
  n29 = global write "RefNums_Actuators.vi" "Upper_Intake"(w64) -> ()
  n30 = call <vilib>:"CTRE_Phoenix_MotorControl_ConfigOpenLoopRamp.vi"("secondsFromNeutralToFull"=0.0, "PhoenixMotorControlDevRef"=w62) -> ()  [unwired: 8 in, 2 out]
  n31 = call <vilib>:"CTRE_Phoenix_MotorControl_ConfigOpenLoopRamp.vi"("secondsFromNeutralToFull"=0.1, "PhoenixMotorControlDevRef"=w63) -> ()  [unwired: 8 in, 2 out]
  n32 = call <vilib>:"WPI_JoystickRefNum Registry Set.vi"("refnum name"=w141, "JoystickDevRef"=w140) -> ()  [unwired: 8 in, 2 out]
  n33 = global write "Joystick RefNum.vi" "Joystick_1"(w141) -> ()
  n34 = call-poly <vilib>:"NT Write Value.vi"("String Array"=string[] ["Alternative 1", "Alternative 2"], "Name"="Auto List") -> ()  [unwired: 9 in, 1 out]
  n35 = call-poly <vilib>:"WPI_SolenoidOpen.vi"("Reverse Solenoid Channel"=WPI_SolenoidChannel."Solenoid 1", "Forward Solenoid Channel"=WPI_SolenoidChannel."Solenoid 7", "Pneumatics Control Module (0)"=w22) -> ("SolenoidDevRef"=w38:T30)  [unwired: 7 in, 1 out]
  n36 = call-poly <vilib>:"WPI_SolenoidOpen.vi"("Reverse Solenoid Channel"=WPI_SolenoidChannel."Solenoid 6", "Forward Solenoid Channel"=WPI_SolenoidChannel."Solenoid 2", "Pneumatics Control Module (0)"=w22) -> ("SolenoidDevRef"=w31:T30)  [unwired: 7 in, 1 out]
  n37 = call-poly <vilib>:"WPI_SolenoidOpen.vi"("Reverse Solenoid Channel"=WPI_SolenoidChannel."Solenoid 6", "Forward Solenoid Channel"=WPI_SolenoidChannel."Solenoid 7", "Pneumatics Control Module (0)"=w1) -> ("SolenoidDevRef"=w54:T30)  [unwired: 7 in, 1 out]
  n38 = call-poly <vilib>:"WPI_SolenoidOpen.vi"("Reverse Solenoid Channel"=WPI_SolenoidChannel."Solenoid 4", "Forward Solenoid Channel"=WPI_SolenoidChannel."Solenoid 5", "Pneumatics Control Module (0)"=w2) -> ("SolenoidDevRef"=w46:T30)  [unwired: 7 in, 1 out]
  n39 = call-poly <vilib>:"WPI_SolenoidOpen.vi"("Reverse Solenoid Channel"=WPI_SolenoidChannel."Solenoid 5", "Forward Solenoid Channel"=WPI_SolenoidChannel."Solenoid 3", "Pneumatics Control Module (0)"=w22) -> ("SolenoidDevRef"=w27:T30)  [unwired: 7 in, 1 out]
  n40 = call-poly <vilib>:"WPI_SolenoidOpen.vi"("Reverse Solenoid Channel"=WPI_SolenoidChannel."Solenoid 5", "Forward Solenoid Channel"=WPI_SolenoidChannel."Solenoid 2") -> ("SolenoidDevRef"=w25:T30)  [unwired: 8 in, 1 out]
  n41 = call-poly <vilib>:"WPI_SolenoidOpen.vi"("Reverse Solenoid Channel"=WPI_SolenoidChannel."Solenoid 5", "Forward Solenoid Channel"=WPI_SolenoidChannel."Solenoid 2") -> ("SolenoidDevRef"=w42:T30)  [unwired: 8 in, 1 out]
  n42 = call-poly <vilib>:"WPI_SolenoidOpen.vi"("Solenoid Channel"=WPI_SolenoidChannel."Solenoid 3" ("Forward Solenoid Channel"), "Pneumatics Control Module (0)"=w2) -> ("SolenoidDevRef"=w39:T30)  [unwired: 8 in, 1 out]
  n43 = call <vilib>:"WPI_CompressorOpen.vi"("Pneumatics Control Module (0)"=w1) -> ("CompressorDevRef"=w56:T31)  [unwired: 13 in, 1 out]
  n44 = call <vilib>:"WPI_CompressorStart.vi"("CompressorDevRef"=w56) -> ("CompressorDevRef"=w55:T31)  [unwired: 9 in, 1 out]
  n45 = call <vilib>:"WPI_SolenoidRefNum Registry Set.vi"("refnum name"=w35, "SolenoidDevRef"=w38) -> ()  [unwired: 8 in, 2 out]
  n46 = call <vilib>:"WPI_SolenoidRefNum Registry Set.vi"("refnum name"=w33, "SolenoidDevRef"=w31) -> ()  [unwired: 8 in, 2 out]
  n47 = disable-structure shown="Disabled" {
    frame Disabled {
      n48 = global write "CurrentMonitoring.vi" "Elevator_1_PDP"(i8 14 ("Upper_Intake_PDP")) -> ()
      n49 = global write "CurrentMonitoring.vi" "Elevator_2_PDP"(i8 15 ("Elevator_2_PDP")) -> ()
      n50 = global write "CurrentMonitoring.vi" "Elevator_3_PDP"(i8 1 ("Elevator_3_PDP")) -> ()
      n51 = global write "CurrentMonitoring.vi" "Elevator_4_PDP"(i8 0 ("Elevator_4_PDP")) -> ()
    }
    frame Enabled {
    }
  }
  n52 = call <vilib>:"WPI_SolenoidRefNum Registry Set.vi"("refnum name"=w51, "SolenoidDevRef"=w54) -> ()  [unwired: 8 in, 2 out]
  n53 = call <vilib>:"WPI_SolenoidRefNum Registry Set.vi"("refnum name"=w48, "SolenoidDevRef"=w46) -> ()  [unwired: 8 in, 2 out]
  n54 = call <vilib>:"WPI_SolenoidRefNum Registry Set.vi"("refnum name"=w29, "SolenoidDevRef"=w27) -> ()  [unwired: 8 in, 2 out]
  n55 = call <vilib>:"WPI_SolenoidRefNum Registry Set.vi"("refnum name"=w26, "SolenoidDevRef"=w25) -> ()  [unwired: 8 in, 2 out]
  n56 = call <vilib>:"WPI_SolenoidRefNum Registry Set.vi"("refnum name"=w44, "SolenoidDevRef"=w42) -> ()  [unwired: 8 in, 2 out]
  n57 = call <vilib>:"WPI_SolenoidRefNum Registry Set.vi"("refnum name"=w41, "SolenoidDevRef"=w39) -> ()  [unwired: 8 in, 2 out]
  n58 = global write "RefNums_Actuators.vi" "Butterfly_Pneumatic"(w51) -> ()
  n59 = global write "RefNums_Actuators.vi" "Climber_Mantis"(w26) -> ()
  n60 = global write "RefNums_Actuators.vi" "Cargo_Arm"(w35) -> ()
  n61 = global write "RefNums_Actuators.vi" "Hatch_Arm"(w33) -> ()
  n62 = global write "RefNums_Actuators.vi" "Hatch_Eject"(w29) -> ()
  n63 = call <vilib>:"WPI_CompressorRefNum Registry Set.vi"("refnum name"=w50, "CompressorDevRef"=w55) -> ()  [unwired: 8 in, 2 out]
  n64 = global write "RefNums_Actuators.vi" "Upper_Pulse"(w41) -> ()
  n65 = call <vilib>:"CTRE_Phoenix_TalonSRX_Open.vi"("Invert"=TRUE, "Device Number"=w103) -> ("CAN Talon SRX Ref"=w88:T23)  [unwired: 8 in, 1 out]
  n66 = call <vilib>:"CTRE_Phoenix_TalonSRX_Open.vi"("Invert"=TRUE, "Device Number"=w93) -> ("CAN Talon SRX Ref"=w87:T23)  [unwired: 8 in, 1 out]
  n67 = call <vilib>:"CTRE_Phoenix_TalonSRX_Open.vi"("Invert"=TRUE, "Device Number"=w91) -> ("CAN Talon SRX Ref"=w89:T23)  [unwired: 8 in, 1 out]
  n68 = global write "RefNums_Actuators.vi" "Shifters"(w48) -> ()
  n69 = global write "RefNums_Actuators.vi" "Compressor"(w50) -> ()
  n70 = call <vilib>:"Spark MAX Open.vi"("Invert"=w106, "Device Number"=w135) -> ("MotorControlDeviceRef"=w138:T23)  [unwired: 8 in, 1 out]
  n71 = call <vilib>:"Spark MAX Open.vi"("Invert"=w106, "Device Number"=w131) -> ("MotorControlDeviceRef"=w133:T23)  [unwired: 8 in, 1 out]
  n72 = call <vilib>:"Spark MAX Open.vi"("Invert"=w111, "Device Number"=w126) -> ("MotorControlDeviceRef"=w128:T23)  [unwired: 8 in, 1 out]
  n73 = call <vilib>:"Spark MAX Open.vi"("Invert"=w111, "Device Number"=w120) -> ("MotorControlDeviceRef"=w122:T23)  [unwired: 8 in, 1 out]
  n74 = call <vilib>:"Spark MAX Open.vi"("Invert"=w106, "Device Number"=w108) -> ("MotorControlDeviceRef"=w110:T23)  [unwired: 8 in, 1 out]
  n75 = call <vilib>:"Spark MAX Open.vi"("Invert"=w111, "Device Number"=w113) -> ("MotorControlDeviceRef"=w115:T23)  [unwired: 8 in, 1 out]
  n76 = global write "RefNums_Actuators.vi" "PTO"(w44) -> ()
  n77 = call <vilib>:"Spark MAX Set Idle Mode.vi"("Idle Mode"=w124, "MotorControlDeviceRef in"=w138) -> ("MotorControlDeviceRef out"=w137:T23)  [unwired: 8 in, 1 out]
  n78 = call <vilib>:"Spark MAX Set Idle Mode.vi"("Idle Mode"=w116, "MotorControlDeviceRef in"=w133) -> ("MotorControlDeviceRef out"=w132:T23)  [unwired: 8 in, 1 out]
  n79 = call <vilib>:"Spark MAX Set Idle Mode.vi"("Idle Mode"=w124, "MotorControlDeviceRef in"=w128) -> ("MotorControlDeviceRef out"=w127:T23)  [unwired: 8 in, 1 out]
  n80 = call <vilib>:"Spark MAX Set Idle Mode.vi"("Idle Mode"=w116, "MotorControlDeviceRef in"=w122) -> ("MotorControlDeviceRef out"=w121:T23)  [unwired: 8 in, 1 out]
  n81 = call <vilib>:"Spark MAX Set Idle Mode.vi"("MotorControlDeviceRef in"=w110) -> ("MotorControlDeviceRef out"=w109:T23)  [unwired: 9 in, 1 out]
  n82 = call <vilib>:"Spark MAX Set Idle Mode.vi"("MotorControlDeviceRef in"=w115) -> ("MotorControlDeviceRef out"=w114:T23)  [unwired: 9 in, 1 out]
  n83 = call <vilib>:"CTRE_Phoenix_MotorControl_SetNeutralMode.vi"("Motor Control Neutral Mode"=CTRE_Phoenix_MotorControl_NeutralMode."Override to Coast", "PhoenixMotorControlDevRef"=w88) -> ("PhoenixMotorControlDevRef"=w101:T23)  [unwired: 8 in, 1 out]
  n84 = global write "CurrentMonitoring.vi" "Upper_Intake_PDP"(i8 7 ("Elevator_4_PDP")) -> ()
  n85 = global write "CurrentMonitoring.vi" "Lower_Intake_PDP"(i8 0 ("Elevator_4_PDP")) -> ()
  n86 = call <vilib>:"CTRE_Phoenix_MotorControl_RefNumRegistrySet.vi"("refnum name"=w86, "PhoenixMotorControlDevRef"=w87) -> ()  [unwired: 8 in, 2 out]
  n87 = global write "RefNums_Actuators.vi" "Elevator_Limit_Switches"(w86) -> ()
  n88 = call <vilib>:"CTRE_Phoenix_MotorControl_Follow.vi"("Master Controller to Follow"=w88, "PhoenixMotorControlDevRef"=w87) -> ()  [unwired: 8 in, 2 out]
  n89 = call <vilib>:"CTRE_Phoenix_MotorControl_Follow.vi"("Master Controller to Follow"=w88, "PhoenixMotorControlDevRef"=w89) -> ()  [unwired: 8 in, 2 out]
  n90 = call <vilib>:"Spark MAX Set Ramp Rate.vi"("Seconds from neutral to full (0)"=w117, "MotorControlDeviceRef in"=w137) -> ("MotorControlDeviceRef"=w136:T23)  [unwired: 8 in, 1 out]
  n91 = call <vilib>:"Spark MAX Set Ramp Rate.vi"("Seconds from neutral to full (0)"=w117, "MotorControlDeviceRef in"=w132) -> ("MotorControlDeviceRef"=w130:T23)  [unwired: 8 in, 1 out]
  n92 = call <vilib>:"Spark MAX Set Ramp Rate.vi"("Seconds from neutral to full (0)"=w117, "MotorControlDeviceRef in"=w127) -> ("MotorControlDeviceRef"=w125:T23)  [unwired: 8 in, 1 out]
  n93 = call <vilib>:"Spark MAX Set Ramp Rate.vi"("Seconds from neutral to full (0)"=w117, "MotorControlDeviceRef in"=w121) -> ("MotorControlDeviceRef"=w119:T23)  [unwired: 8 in, 1 out]
  n94 = call <vilib>:"Spark MAX Set Ramp Rate.vi"("MotorControlDeviceRef in"=w109) -> ("MotorControlDeviceRef"=w107:T23)  [unwired: 9 in, 1 out]
  n95 = call <vilib>:"Spark MAX Set Ramp Rate.vi"("MotorControlDeviceRef in"=w114) -> ("MotorControlDeviceRef"=w112:T23)  [unwired: 9 in, 1 out]
  n96 = call <vilib>:"CTRE_Phoenix_MotorControl_ConfigAllSettingsEnhanced.vi"("timeoutMs"=100, "Enhanced Motor Controller Configurables"="Talon Enhanced Config", "PhoenixMotorControlDevRef"=w101) -> ("PhoenixMotorControlDevRef"=w100:T23)  [unwired: 7 in, 1 out]
  n97 = global write "RefNums_Actuators.vi" "Drive_6R"(w105) -> ()
  n98 = global write "RefNums_Actuators.vi" "Drive_5L"(w104) -> ()
  n99 = global write "RefNums_Actuators.vi" "Drive_2R"(w129) -> ()
  n100 = global write "RefNums_Actuators.vi" "Drive_3L"(w123) -> ()
  n101 = global write "RefNums_Actuators.vi" "Drive_4L"(w118) -> ()
  n102 = global write "RefNums_Actuators.vi" "Drive_1R"(w134) -> ()
  n103 = call <vilib>:"WPI_MotorControlRefNum Registry Set.vi"("refnum name"=w134, "MotorControlDevRef"=w136) -> ()  [unwired: 8 in, 2 out]
  n104 = call <vilib>:"WPI_MotorControlRefNum Registry Set.vi"("refnum name"=w129, "MotorControlDevRef"=w130) -> ()  [unwired: 8 in, 2 out]
  n105 = call <vilib>:"WPI_MotorControlRefNum Registry Set.vi"("refnum name"=w123, "MotorControlDevRef"=w125) -> ()  [unwired: 8 in, 2 out]
  n106 = call <vilib>:"WPI_MotorControlRefNum Registry Set.vi"("refnum name"=w118, "MotorControlDevRef"=w119) -> ()  [unwired: 8 in, 2 out]
  n107 = call <vilib>:"WPI_MotorControlRefNum Registry Set.vi"("refnum name"=w105, "MotorControlDevRef"=w107) -> ()  [unwired: 8 in, 2 out]
  n108 = call <vilib>:"WPI_MotorControlRefNum Registry Set.vi"("refnum name"=w104, "MotorControlDevRef"=w112) -> ()  [unwired: 8 in, 2 out]
  n109 = disable-structure shown="Disabled" {
    frame Disabled {
      w163 = "Right_Prox_Sensor" ("refnum name")
      n110 = call <vilib>:"WPI_AnalogChannelOpen.vi"("Analog Channel"=FPGA_AIChannel."AI 0") -> ("AIDeviceRef"=w165:T32)  [unwired: 9 in, 1 out]
      n111 = call <vilib>:"WPI_AnalogChannelRefNum Registry Set.vi"("refnum name"=w163, "AIDeviceRef"=w165) -> ()  [unwired: 8 in, 2 out]
      n112 = global write "RefNums_Sensors.vi" "Right_Prox_Sensor"(w163) -> ()
    }
    frame Enabled {
    }
  }
  n113 = call <vilib>:"CTRE_Phoenix_MotorControl_RefNumRegistrySet.vi"("refnum name"=w99, "PhoenixMotorControlDevRef"=w100) -> ()  [unwired: 8 in, 2 out]
  n114 = disable-structure shown="Disabled" {
    frame Disabled {
      w166 = "Right_Prox_Sensor" ("refnum name")
      n115 = call <vilib>:"WPI_AnalogChannelOpen.vi"("Analog Channel"=FPGA_AIChannel."AI 1") -> ("AIDeviceRef"=w168:T32)  [unwired: 9 in, 1 out]
      n116 = call <vilib>:"WPI_AnalogChannelRefNum Registry Set.vi"("refnum name"=w166, "AIDeviceRef"=w168) -> ()  [unwired: 8 in, 2 out]
      n117 = global write "RefNums_Sensors.vi" "Right_Prox_Sensor"(w166) -> ()
    }
    frame Enabled {
    }
  }
  n118 = disable-structure shown="Disabled" {
    frame Disabled {
      w169 = "Right_Prox_Sensor" ("refnum name")
      n119 = call <vilib>:"WPI_AnalogChannelOpen.vi"("Analog Channel"=FPGA_AIChannel."AI 2") -> ("AIDeviceRef"=w171:T32)  [unwired: 9 in, 1 out]
      n120 = call <vilib>:"WPI_AnalogChannelRefNum Registry Set.vi"("refnum name"=w169, "AIDeviceRef"=w171) -> ()  [unwired: 8 in, 2 out]
      n121 = global write "RefNums_Sensors.vi" "Right_Prox_Sensor"(w169) -> ()
    }
    frame Enabled {
    }
  }
  n122 = global write "RefNums_Actuators.vi" "Elevator"(w99) -> ()
  n123 = call <vilib>:"WPI_AnalogChannelOpen.vi"("Analog Channel"=FPGA_AIChannel."AI 3") -> ("AIDeviceRef"=w21:T32)  [unwired: 9 in, 1 out]
  n124 = call <vilib>:"WPI_AnalogChannelOpen.vi"("Analog Channel"=FPGA_AIChannel."AI MXP 0") -> ("AIDeviceRef"=w18:T32)  [unwired: 9 in, 1 out]
  n125 = call <vilib>:"WPI_AnalogChannelOpen.vi"("Analog Channel"=FPGA_AIChannel."AI MXP 1") -> ("AIDeviceRef"=w15:T32)  [unwired: 9 in, 1 out]
  n126 = call <vilib>:"WPI_AnalogChannelOpen.vi"("Analog Channel"=FPGA_AIChannel."AI MXP 2") -> ("AIDeviceRef"=w12:T32)  [unwired: 9 in, 1 out]
  n127 = call <vilib>:"WPI_AnalogChannelOpen.vi"("Analog Channel"=FPGA_AIChannel."AI MXP 3") -> ("AIDeviceRef"=w9:T32)  [unwired: 9 in, 1 out]
  n128 = call-poly <vilib>:"WPI_AccelerometerOpen.vi"("Accel Range"=WPI_AccelerometerRange."+/- 2 g") -> ("error out"=w4:errorcluster, "AccelerometerDevRef"=w6:T33)  [unwired: 9 in]
  n129 = global write "RefNums_Sensors.vi" "Upper_Pressure_Transducer"(w19) -> ()
  n130 = global write "RefNums_Sensors.vi" "Tank_Pressure_Transducer"(w7) -> ()
  n131 = call <vilib>:"WPI_AnalogChannelRefNum Registry Set.vi"("refnum name"=w19, "AIDeviceRef"=w21) -> ()  [unwired: 8 in, 2 out]
  n132 = call <vilib>:"WPI_AnalogChannelRefNum Registry Set.vi"("refnum name"=w16, "AIDeviceRef"=w18) -> ()  [unwired: 8 in, 2 out]
  n133 = global write "RefNums_Sensors.vi" "Front_Right_Prox_Sensor"(w16) -> ()
  n134 = call <vilib>:"WPI_AnalogChannelRefNum Registry Set.vi"("refnum name"=w13, "AIDeviceRef"=w15) -> ()  [unwired: 8 in, 2 out]
  n135 = call <vilib>:"WPI_AnalogChannelRefNum Registry Set.vi"("refnum name"=w10, "AIDeviceRef"=w12) -> ()  [unwired: 8 in, 2 out]
  n136 = call <vilib>:"WPI_AnalogChannelRefNum Registry Set.vi"("refnum name"=w7, "AIDeviceRef"=w9) -> ()  [unwired: 8 in, 2 out]
  n137 = global write "RefNums_Sensors.vi" "Front_Left_Prox_Sensor"(w13) -> ()
  n138 = global write "RefNums_Sensors.vi" "Ground_Prox_Sensor"(w10) -> ()
  n139 = global write "RefNums_Sensors.vi" "Accelerometer"(w3) -> ()
  n140 = call <vilib>:"WPI_AccelerometerRefNum Registry Set.vi"("error in (no error)"=w4, "refnum name"=w3, "AccelerometerDevRef"=w6) -> ()  [unwired: 7 in, 2 out]
  "error out" <- "error in"
